vi "Read DAQ Queue.vi"(8 "error in (no error)":errorcluster, 11 "DAQ Interface in":refnum<class "DAQ Interface.lvclass">) -> (0 "error out":errorcluster, 2 "DAQ Queue":refnum<queue>, 3 "DAQ Interface out":refnum<class "DAQ Interface.lvclass">)   [LabVIEW 2020, in "DAQ Interface.lvlib" / "DAQ Interface.lvclass"]
uses:
  DAQ Interface.lvclass
  Signal Analysis/Signal Analysis/Process Data.ctl
  <vilib>/Natan Biesmans/G2CPU GPU and CPU HPC Toolkit/G2CPU Libraries/Arrays/1DArray/s16/1D Array s16.lvclass
  DAQ Interface.lvclass/DAQ Interface.ctl
  Signal Analysis/Signal Analysis/Signal Analysis.lvclass
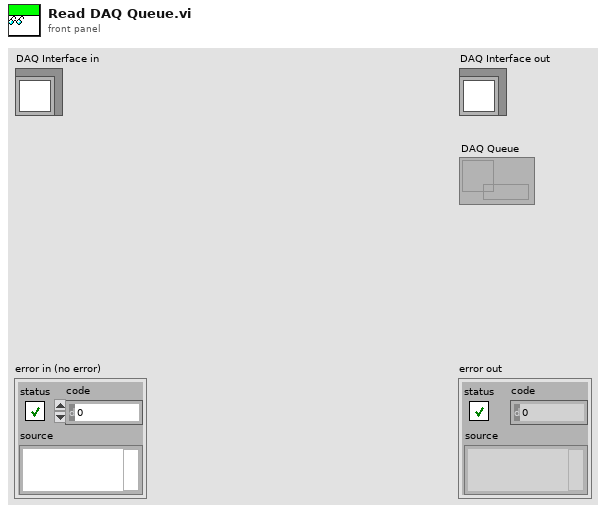
[diagram p1: front panel]
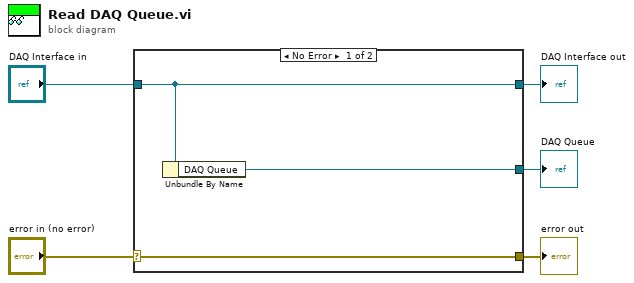
[diagram p0: block diagram]
diagram:
  n1 = case shown="No Error" "error in (no error)" {
    selector: "error in (no error)" -> [w8 w9]
    tunnel: [w8 w9] -> w4
    tunnel: [w7 w10] -> w2
    tunnel: "DAQ Interface in" -> [w7 w10]
    tunnel: [w6 _] -> w1
    frame No Error {
      n2 = Unbundle By Name(w7) -> ("DAQ Queue"=w6:refnum<queue>)
    }
    frame Error {
    }
  }
  "error out" <- w4
  "DAQ Interface out" <- w2
  "DAQ Queue" <- w1
